vi "tsdiag_can_delete_all.vi"(8 "错误输入（无错误）":errorcluster, 11 "path":path) -> (0 "错误输出":errorcluster, 2 "return":i32, 3 "path out":path)   [LabVIEW 2014]
doc: "Function Introduction :\nDelete all CAN UDS diagnostic services\nCall location :\ninput parameter :\nnothing\nReturn value :\n==0: Execution successful\nOther values: Query error code"
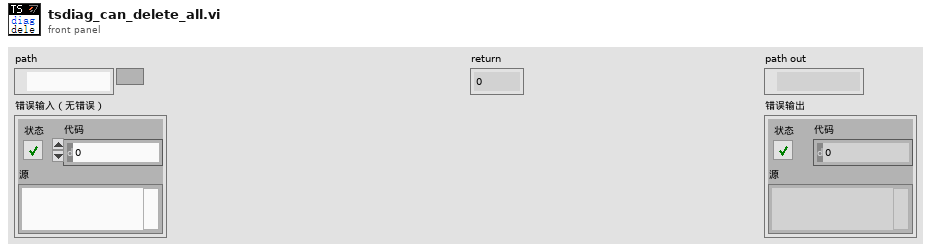
[diagram p1: front panel]
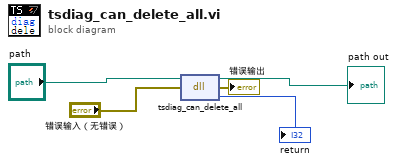
[diagram p0: block diagram]
diagram:
  n1 = dll-call lib="C:/Users/XYY/Desktop/LabView Demo/TSCAN_LB2018_V1.4_20220309/Config/TSMaster.dll" fn="tsdiag_can_delete_all"(path in="path", error in="错误输入（无错误）") -> (path out=→"path out":path, error out=→"错误输出":errorcluster, "return"=→"return":i32)  [unwired: 1 in]
